vi "Flatten.vi"(8 "error in":errorcluster, 9 "Data":T1) -> (0 "error out":errorcluster, 2 "Buffer":u8[](array[numeric]) format="%.0x")   [LabVIEW 2020, in "RequestTwoDouble.lvlib"]
uses:
  RequestTwoDouble.lvlib
  Data.ctl
  lv-protoc/LV-Proto/LV-Proto.lvlib
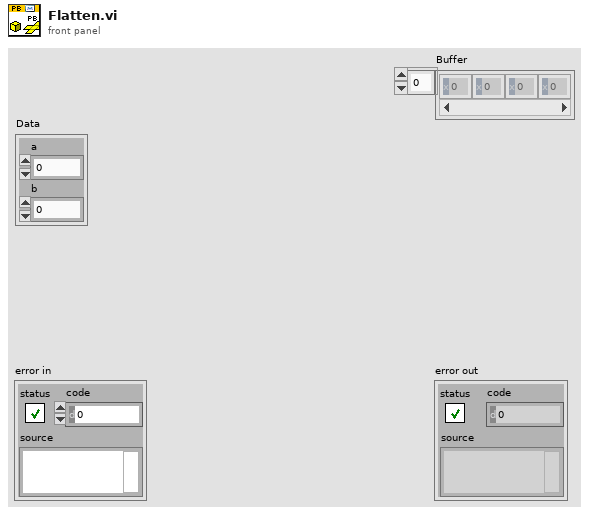
[diagram p1: front panel]
types:
  T1 = typedef "RequestTwoDouble.lvlib/Data.ctl" = cluster{"a":dbl, "b":dbl}
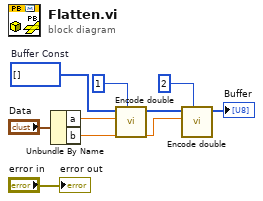
[diagram p0: block diagram]
diagram:
  w7 = u8[] []  # Buffer Const
  n1 = Unbundle By Name("Data") -> ("a"=w5:dbl, "b"=w2:dbl)
  n2 = call "Encode double.vi"("Field Number"=1, "double"=w5, "Buffer in"=w7) -> ("Buffer"=w4:u8[])  [unwired: 8 in]
  n3 = call "Encode double.vi"("Field Number"=2, "double"=w2, "Buffer in"=w4) -> ("Buffer"=→"Buffer":u8[])  [unwired: 8 in]
  "error out" <- "error in"
